vi "ConvertIntToStr.vi"(11 "data":i32) -> (3 "result":string)   [LabVIEW 2018, in "Library-DataConvert.lvlib"]
uses:
  Library-DataConvert.lvlib
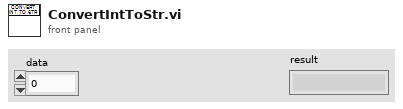
[diagram p1: front panel]
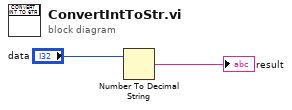
[diagram p0: block diagram]
diagram:
  n1 = Number To Decimal String(number="data") -> (decimal integer string=→"result":string)  [unwired: 1 in]
